vi "cs_usb_close.vi"(2 "error in (no error)":errorcluster, 3 "cs_usb handle":i32) -> (0 "error out":errorcluster, 1 "handle out":i32)   [LabVIEW 2017]
uses:
  kernel32.dll
panel:
  out "handle 2":i32=1
  out "handle":i32=1
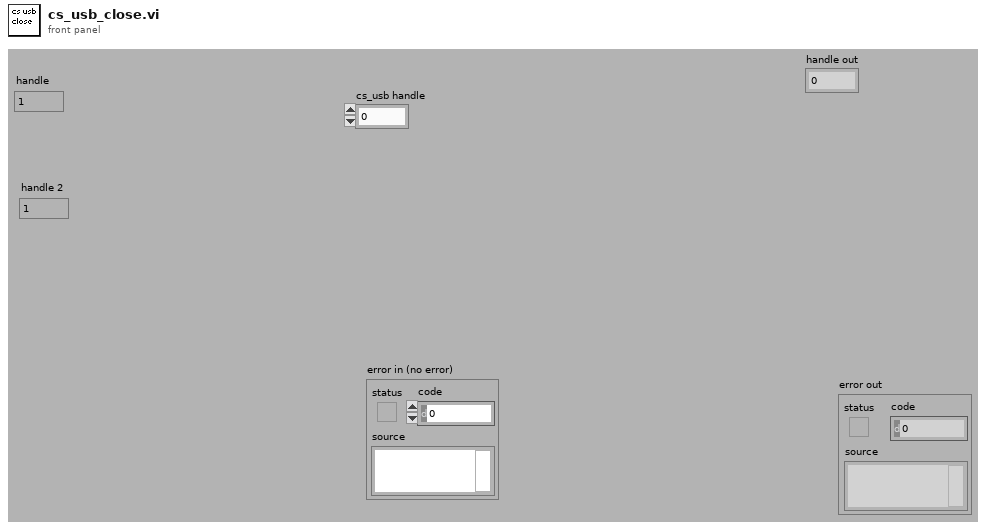
[diagram p1: front panel]
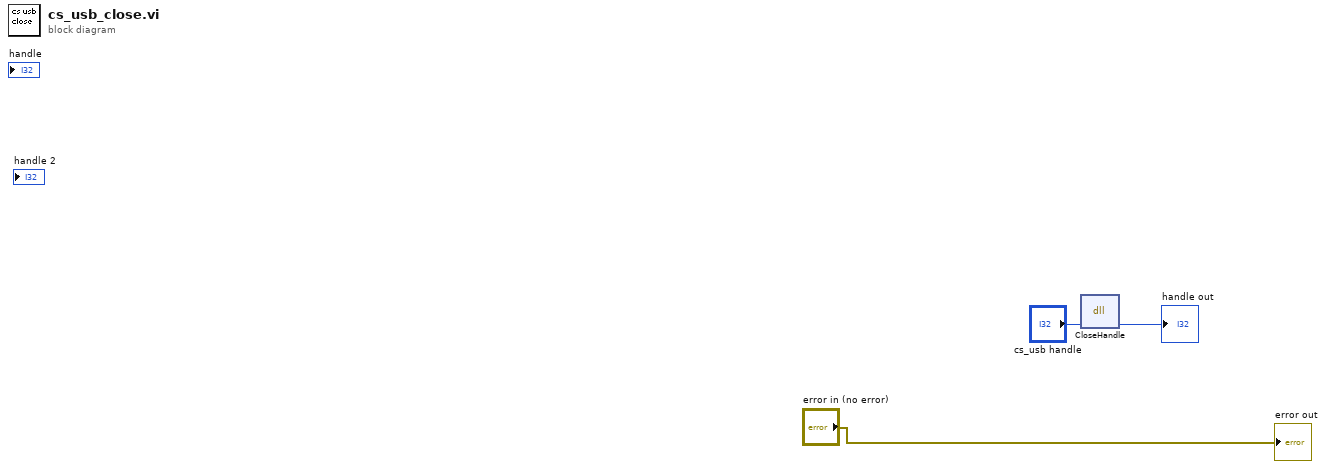
[diagram p0: block diagram]
diagram:
  n1 = dll-call lib="kernel32.dll" fn="CloseHandle"("handle"="cs_usb handle") -> ("handle"=→"handle out":i32)  [unwired: 4 in, 2 out]
  "error out" <- "error in (no error)"
